vi "UV-VIS SetTemperature.vi"(3 "error in (no error)":errorcluster, 4 "temperature":i32=20, 5 "UV-VIS detector in":refnum<class "CCD_camera.lvclass">) -> (0 "error out":errorcluster, 1 "DLL error code":u32, 2 "UV-VIS detector out":refnum<class "CCD_camera.lvclass">)   [LabVIEW 2020, in "CCD_camera.lvclass"]
doc: "This function will set the desired temperature of the detector. To turn the cooling ON and OFF use the <B>CoolerON</B> and <B>CoolerOFF</B> function respectively.\n\n<B>Parameters:</B>\ntemperature - the temperature in Centigrade.\n Valid range is given by <B>GetTemperatureRange</B>\n\n<B>Error codes:</B>\nDRV_SUCCESS - Accumulations set.\nDRV_NOT_INITIALIZED - System not initialized.\nDRV_ACQUIRING - Acquisition in progress.\nDRV_ERROR_ACK - Unable to communicate with card.\nDRV_P1INVALID - Temperature invalid."
uses:
  CCD_camera.lvclass
  C:/dev/TRANCON/Classes/Detector/Detector.lvclass
  C:/dev/TRANCON/Classes/GeneralFunctionality/GeneralFunctionality.lvclass
  Detector.lvclass/Detector.ctl
  GeneralFunctionality/GeneralFunctionality.lvclass/GeneralFunctionality.ctl
  Config/Config.lvclass
  Detector.lvclass
  GeneralFunctionality/GeneralFunctionality.lvclass
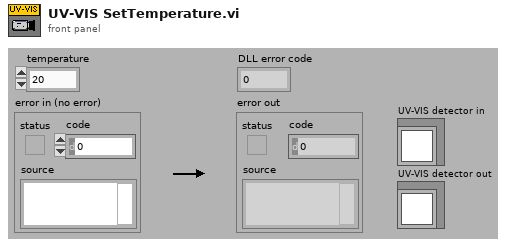
[diagram p1: front panel]
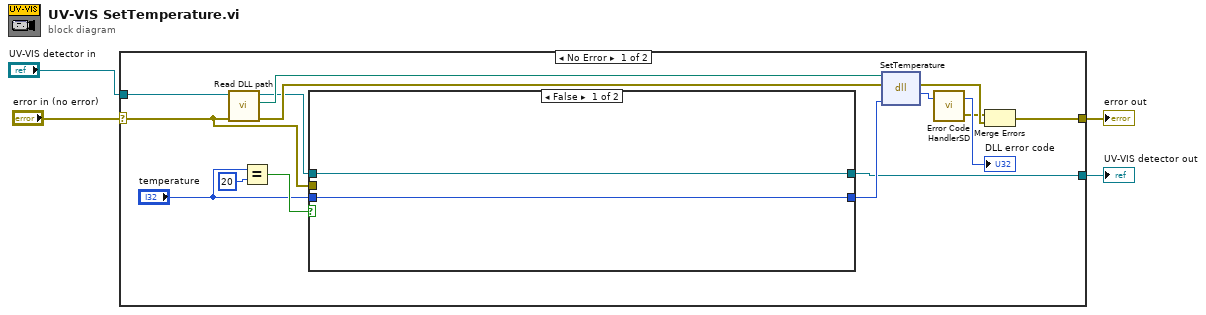
[diagram p0: block diagram]
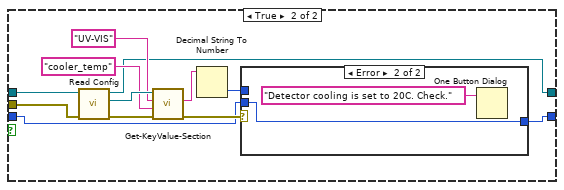
[diagram p2: hidden frame]
diagram:
  n1 = case shown="No Error" "error in (no error)" {
    selector: "error in (no error)" -> [w9 w38]
    tunnel: [w13 w38] -> w3
    tunnel: [w5 w37] -> w2
    tunnel: "UV-VIS detector in" -> [w10 w37]
    frame No Error {
      n2 = call "Read DLL path.vi"("error in (no error)"=w9, "Detector in"=w10) -> ("error out"=w16:errorcluster, "DLL path"=w17:path, "Detector out"=w6:refnum<class "CCD_camera.lvclass">)  [unwired: 7 in]
      n3 = Equal?(x="temperature", y=20) -> (x = y?=w11:bool)
      n4 = case shown="False" w11 {
        tunnel: w6 -> [w20 w29]
        tunnel: w9 -> [_ w27]
        tunnel: [w21 w25] -> w7
        tunnel: "temperature" -> [w21 w24]
        tunnel: [w20 w22] -> w5
        frame False {
        }
        frame True {
          n5 = call "Read Config.vi"("error in (no error)"=w27, "GeneralFunctionality en entrée"=w29) -> ("error out"=w28:errorcluster, "Config.lvclass"=w33:refnum<class "Config.lvclass">, "GeneralFunctionality en sortie"=w22:refnum<class "CCD_camera.lvclass">)  [unwired: 7 in]
          n6 = call-dynamic "Get-KeyValue-Section.vi"("error in (no error)"=w28, "Key"="cooler_temp", "Section"="UV-VIS", "Config in"=w33) -> ("error out"=w26:errorcluster, "Value"=w30:string)  [unwired: 5 in, 1 out]
          n7 = Decimal String To Number(string=w30) -> (number=w23:i32)  [unwired: 2 in, 1 out]
          n8 = case shown="Error" w26 {
            tunnel: w23 -> [w34 _]
            tunnel: [w34 w36] -> w25
            tunnel: w24 -> [_ w36]
            frame No Error {
            }
            frame Error {
              n9 = One Button Dialog(message="Detector cooling is set to 20C. Check.") -> ()  [unwired: 1 in, 1 out]
            }
          }
        }
      }
      n10 = dll-call lib="S:/TRANCON/DLL/Atmcd32d.dll" fn="SetTemperature"(path in=w17, error in=w16, "temperature"=w7) -> (error out=w15:errorcluster, "return type"=w19:u32)  [unwired: 2 in, 1 out]
      n11 = call "Error Code HandlerSD.vi"("DLL error code"=w19) -> ("error out"=w14:errorcluster, "dup DLL error code"=→"DLL error code":u32)  [unwired: 1 in]
      n12 = Merge Errors(w14, w15) -> (w13:errorcluster)
    }
    frame Error {
    }
  }
  "error out" <- w3
  "UV-VIS detector out" <- w2
